vi "View Model - Init.vi"(8 "error in (no error)":errorcluster) -> (0 "error out":errorcluster, 3 "View Model":T1)   [LabVIEW 2017]
doc: "Initialize all components of View Model container."
uses:
  Controls/View Model.ctl
  Controls/Shared Model.ctl
  Error Handler/Controls/Error Model.ctl
  Error Handler/Controls/Error Data.ctl
  Error Handler/Controls/Error Level.ctl
  Configuration/Controls/Config Model.ctl
  Configuration/Controls/Config Record.ctl
  Configuration/Controls/Config Data.ctl
  Configuration/Controls/Config Command.ctl
  Controller/Controls/Controler Model.ctl
  Views/Entry Console View/Controls/Entry Console - Wash Steps.ctl
  Controller/Controls/Controller - Overhead.ctl
  Controller/Controls/Controller - States.ctl
  Controller/Controls/Controller - Wash Step.ctl
  Views/Vehicle Position View/Controls/Vehicle - Station Enum.ctl
  Controller/Controls/Controller - Event.ctl
  Controller/Controls/Controller - Commands.ctl
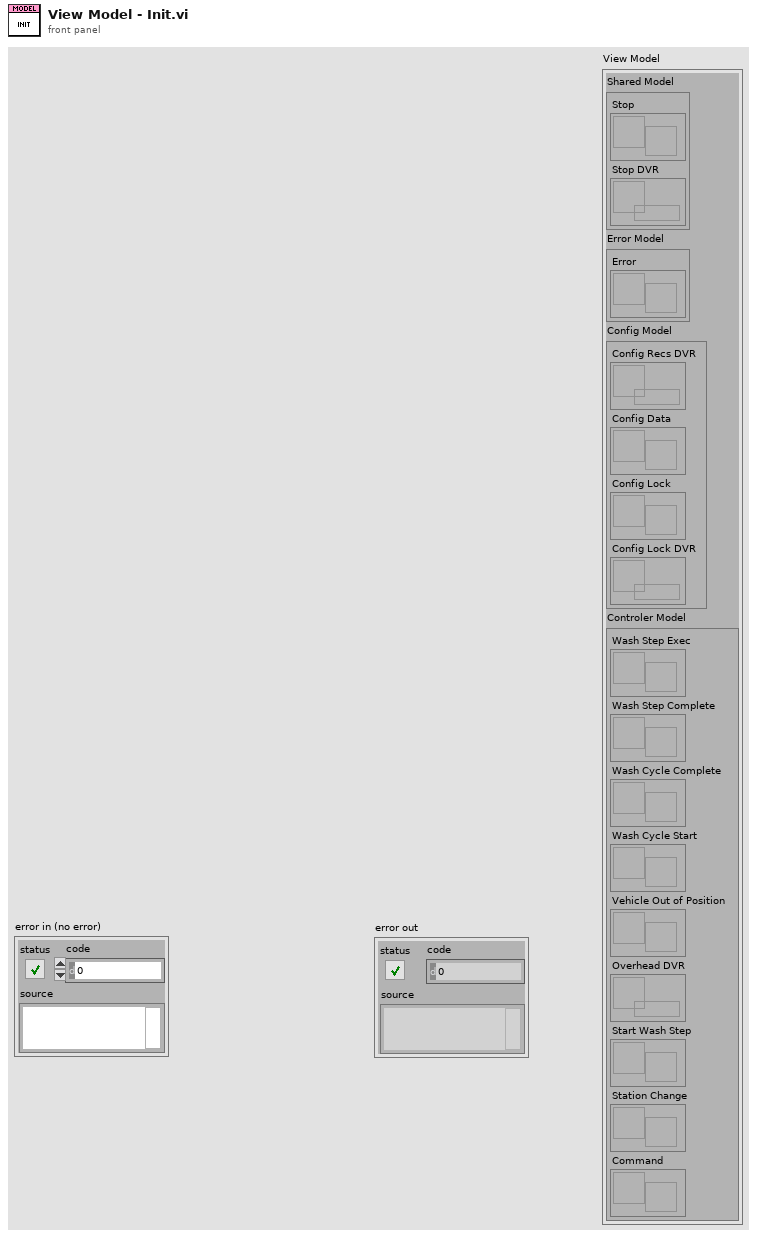
[diagram p1: front panel]
types:
  T1 = typedef "View Model.ctl" = cluster{"Shared Model":T2, "Error Model":T3, "Config Model":T4, "Controler Model":T5}
  T2 = typedef "Shared Model.ctl" = cluster{"Stop":refnum<user-event>, "Stop DVR":refnum<data-value>}
  T3 = typedef "Error Model.ctl" = cluster{"Error":refnum<user-event>}
  T4 = typedef "Config Model.ctl" = cluster{"Config Recs DVR":refnum<data-value>, "Config Data":refnum<user-event>, "Config Lock":refnum<user-event>, "Config Lock DVR":refnum<data-value>}
  T5 = typedef "Controler Model.ctl" = cluster{"Wash Step Exec":refnum<user-event>, "Wash Step Complete":refnum<user-event>, "Wash Cycle Complete":refnum<user-event>, "Wash Cycle Start":refnum<user-event>, "Vehicle Out of Position":refnum<user-event>, "Overhead DVR":refnum<data-value>, "Start Wash Step":refnum<user-event>, "Station Change":refnum<user-event>, "Command":refnum<user-event>}
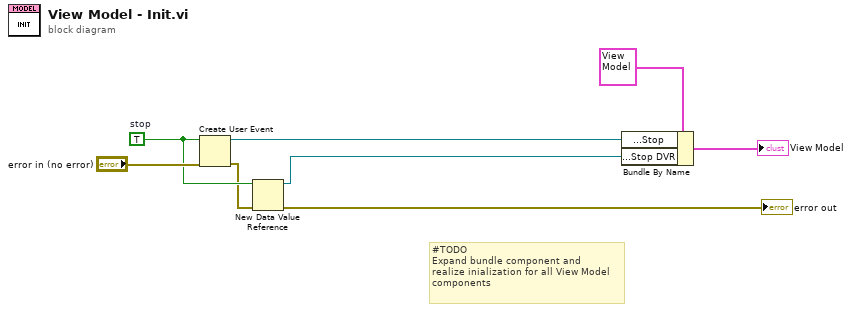
[diagram p0: block diagram]
diagram:
  w5 = TRUE  # stop
  # "#TODO\nExpand bundle component and\nrealize inialization for all View Model\ncomponents"
  n1 = Create User Event(user event datatype=w5, error in="error in (no error)") -> (user event=w3:refnum<user-event>, error out=w4:errorcluster)
  n2 = New Data Value Reference(data value=w5, error in=w4) -> (data value reference=w2:refnum<data-value>, error out=→"error out":errorcluster)
  n3 = Bundle By Name(cluster=T1 {"Shared Model"={"Stop"=refnum, "Stop DVR"=refnum}, "Error Model"={"Error"=refnum}, "Config Model"={"Config Recs DVR"=refnum, "Config Data"=refnum, "Config Lock"=refnum, "Config Lock DVR"=refnum}, "Controler Model"={"Wash Step Exec"=refnum, "Wash Step Complete"=refnum, "Wash Cycle Complete"=refnum, "Wash Cycle Start"=refnum, "Vehicle Out of Position"=refnum, "Overhead DVR"=refnum, "Start Wash Step"=refnum, "Station Change"=refnum, "Command"=refnum}} ("View Model"), "Shared Model.Stop"=w3, "Shared Model.Stop DVR"=w2) -> (→"View Model":T1)
